vi "Build MD5 Hash Code.vi"(6 "Assert VI Path":path, 8 "error in (no error)":errorcluster, 11 "Test in":refnum<class "Test.lvclass">) -> (0 "error out":errorcluster, 3 "Test out":refnum<class "Test.lvclass">)   [LabVIEW 2018, in "Test.lvclass"]
uses:
  Test.lvclass
  Test Class String IDs.vi
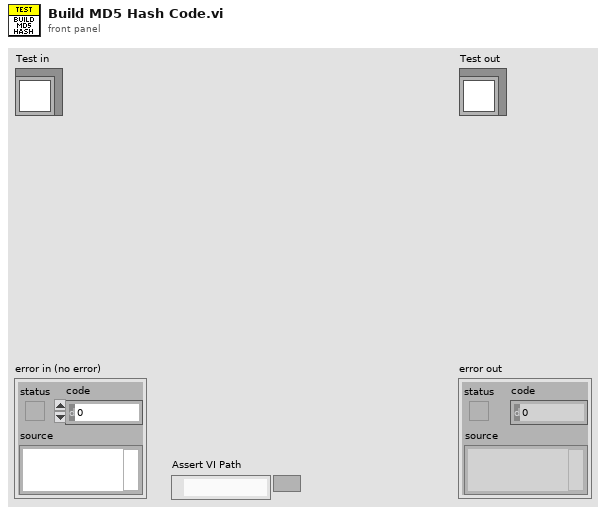
[diagram p1: front panel]
types:
  T1 = cluster{"Comparison Value 1":string, "Comparison Value 2":string, "Invert Result":string, "Assert VI Name":string, "Data Type":string, "Builder User Name":string, "Build Timestamp":string, "Failure Action":string, "Comment":string, "Assert Name":string, "Description":string, "Evaluation String":string, "MD5":string}
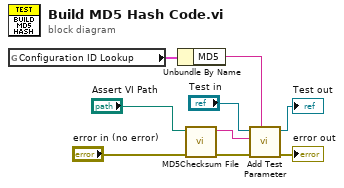
[diagram p0: block diagram]
diagram:
  n1 = global read "Test Class String IDs.vi" "Configuration ID Lookup"() -> (w6:T1)
  n2 = Unbundle By Name(w6) -> ("MD5"=w5:string)
  n3 = call <vilib>:"MD5Checksum File.vi"("error in (no error)"="error in (no error)", "Path"="Assert VI Path") -> ("error out"=w3:errorcluster, "MD5 message-digest"=w4:string)  [unwired: 8 in]
  n4 = call-dynamic "Add Test Parameter.vi"("Data Value ID"=w5, "error in (no error)"=w3, "Data Value"=w4, "Test in"="Test in") -> ("error out"=→"error out":errorcluster, "Test out"=→"Test out":refnum<class "Test.lvclass">)  [unwired: 5 in, 1 out]
